vi "Message Handling Loop - File IO.vi"(8 "error in":errorcluster, 9 "Message Queues in":T1, 10 "User Event Bundle":T2) -> (0 "error out":errorcluster)   [LabVIEW 2018]
uses:
  Type Defs/User Events.ctl
  Support/Message Queue/All Message Queues.ctl
  Support/Message Queue/Message Cluster.ctl
  Type Defs/File IO Loop Data.ctl
  Type Defs/FGV States.ctl
  Support/Message Queue/Enqueue Message (Single).vi
  <vilib>/Utility/error.llb/Error Cluster From Error Code.vi
  <vilib>/ErrorRing/Error Ring.xnode
  Support/Message Queue/Message Queue.lvlib
  Support/User Events/User Events.lvlib
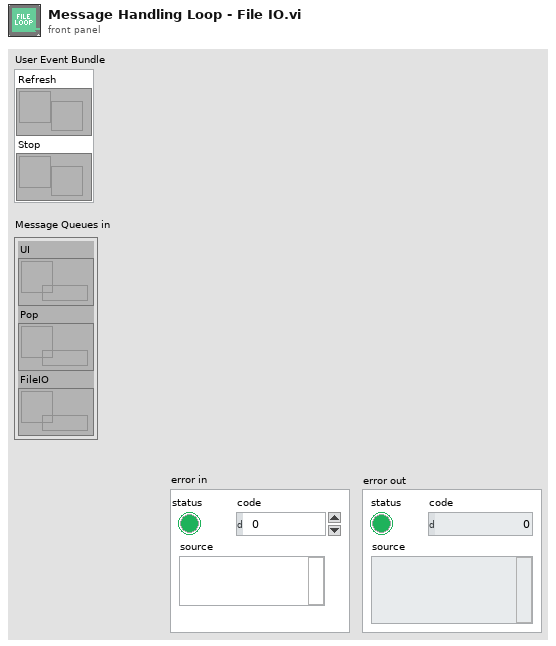
[diagram p1: front panel]
types:
  T1 = typedef "Message Queue.lvlib/All Message Queues.ctl" = cluster{"UI":refnum<queue>, "Pop":refnum<queue>, "FileIO":refnum<queue>}
  T2 = typedef "User Events.ctl" = cluster{"Refresh":refnum<user-event>, "Stop":refnum<user-event>}
  T3 = typedef "File IO Loop Data.ctl" = cluster{"Data Folder File Path":path, "UI":refnum<queue>, "Pop":refnum<queue>, "FileIO":refnum<queue>, "Open Notes":i32[], "Main VI":refnum<vi>, "Update Path":path}
  T4 = typedef "FGV States.ctl" = enum16{"Initialize", "Merge", "Write", "Remove", "Read", "Clear"}
  T5 = typedef "SR Cluster.ctl" = cluster{"Color":u32, "SR Number":i32, "SR Status":T6, "Name":string, "Summary":string, "Last Updated":timestamp, "SR Type":string, "Service Level":string, "Days Open":dbl, "Creation Date":timestamp, "Owner":string, "Note":string}
  T6 = typedef "SR Status.ctl" = enum16{"Caller Abandoned", "Created in Error", "Expired", "Forum Resolved AE", "Forum Resolved Customer", "IN WORK", "IN WORK Collab with AES", "IN WORK Collab with PSE", "IN WORK Collab with SE", "IN WORK Customer Added Note", "IN WORK Escalation", "IN WORK Wait on Customer", "Open", "Potentially Resolved", "Presumed Resolved", "RMA Approved for Return", "RMA Closed", "RMA Closed - DOA", "RMA In Progress", "RMA Open", "RMA Waiting on Customer", "Resolved", "Passed Off"}
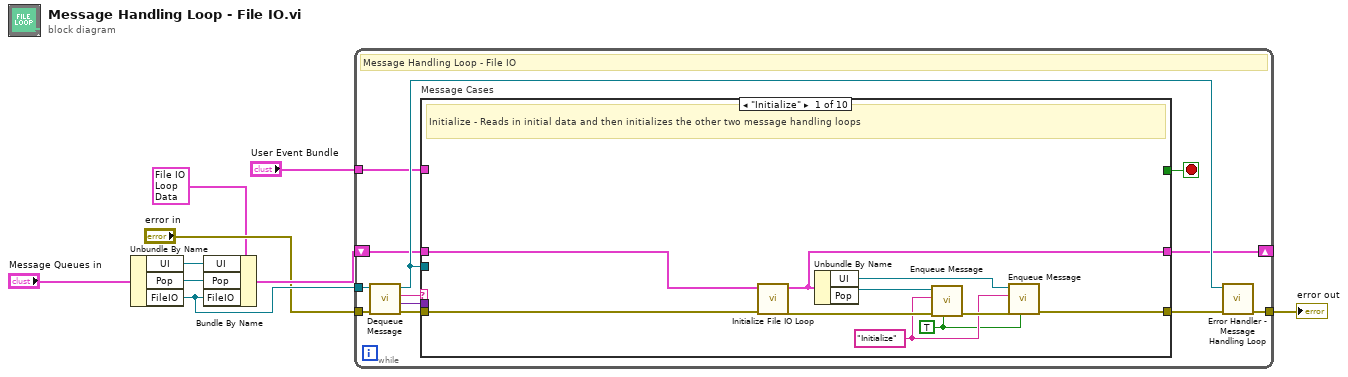
[diagram p0: block diagram]
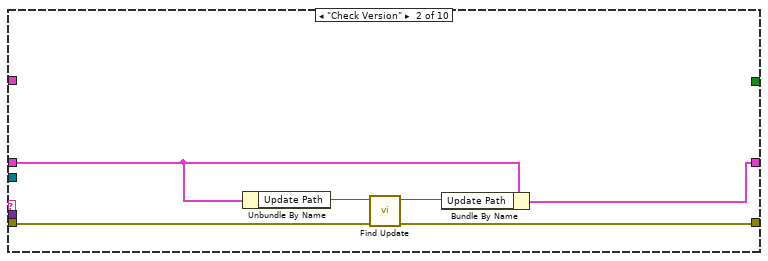
[diagram p2: hidden frame]
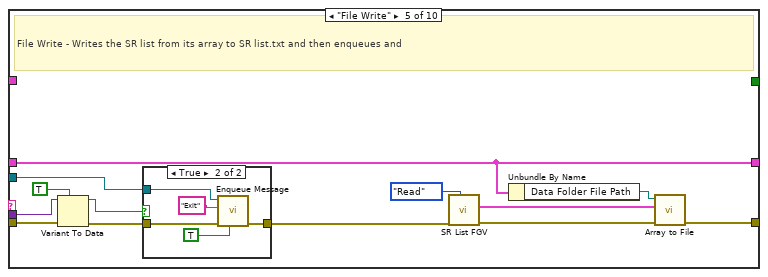
[diagram p5: hidden frame]
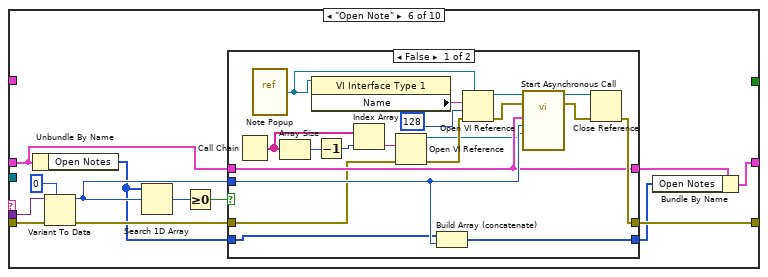
[diagram p7: hidden frame]
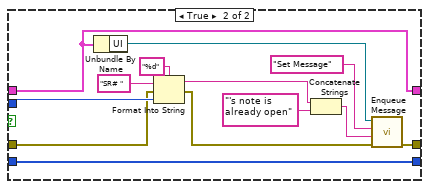
[diagram p8: hidden frame]
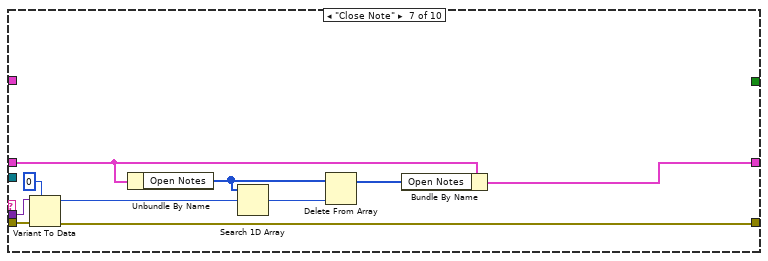
[diagram p9: hidden frame]
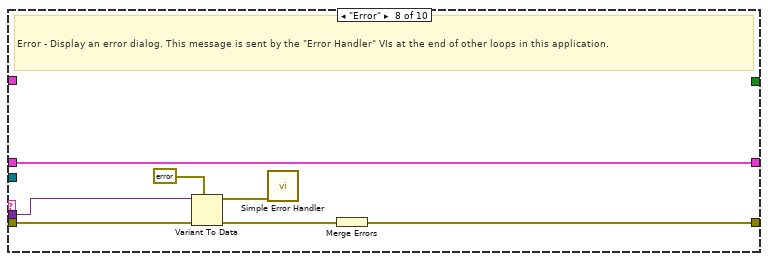
[diagram p10: hidden frame]
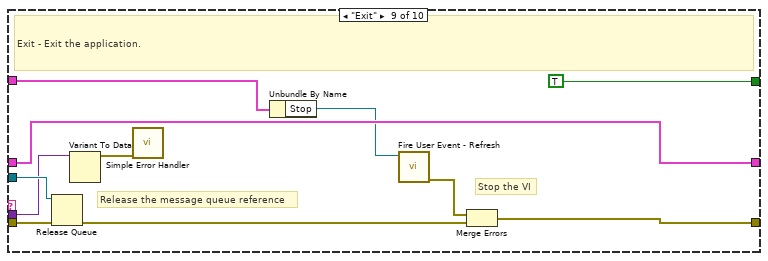
[diagram p11: hidden frame]
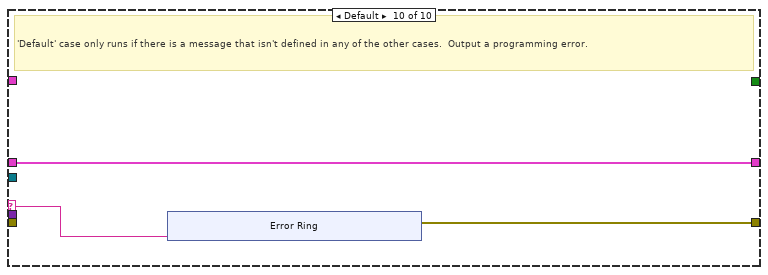
[diagram p12: hidden frame]
diagram:
  n1 = Unbundle By Name("Message Queues in") -> ("UI"=w6:refnum<queue>, "Pop"=w4:refnum<queue>, "FileIO"=w5:refnum<queue>)
  n2 = Bundle By Name(cluster=T3 {"Data Folder File Path"=path "", "UI"=refnum, "Pop"=refnum, "FileIO"=refnum, "Open Notes"=[], "Main VI"=refnum, "Update Path"=path ""} ("Data Loop Data"), "UI"=w6, "Pop"=w4, "FileIO"=w5) -> (w7:T3)
  n3 = while {
    tunnel: w5 -> [w17]
    tunnel: [w15] -> w1
    shift-right: [w12] -> _
    shift-left: w7 -> [w13]
    tunnel: "User Event Bundle" -> [w11]
    tunnel: "error in" -> [w10]
    stop <- w21 stop-if-true
    # "Message Handling Loop - File IO"
    n4 = call "Dequeue Message.vi"("error in (no error)"=w10, "Message Queue"=w17) -> ("error out"=w20:errorcluster, "Message Data"=w18:variant, "Message"=w19:string, "dup Message Queue"=w16:refnum<queue>)  [unwired: 6 in]
    n5 = case "Message Cases" shown="\"Initialize\"" w19 {
      selector: w19 -> [_ _ _ _ _ _ _ _ _ w135]
      tunnel: w16 -> [_ _ _ _ w46 _ _ _ w133 _]
      tunnel: w20 -> [w30 w37 w39 w41 w49 w72 w115 w122 w129 _]
      tunnel: [w25 w36 w39 w41 w50 w70 w112 w117 w130 w136] -> w14
      tunnel: [_ _ _ _ _ _ _ _ TRUE _] -> w21
      tunnel: w18 -> [_ _ _ _ w42 w73 w114 w121 w127 _]
      tunnel: w13 -> [w31 w34 w38 w40 w45 w64 w108 w116 w126 w134]
      tunnel: [w29 w32 w38 w40 w45 w61 w106 w116 w126 w134] -> w12
      tunnel: w11 -> [_ _ _ _ _ _ _ _ w125 _]
      frame "Initialize" {
        w22 = TRUE ("Priority Message? (F)")
        w23 = "Initialize" ("Message")
        # "Initialize - Reads in initial data and then initializes the other two message handling loops"
        n6 = call "Initialize File IO Loop.vi"("error in"=w30, "File Loop Data in"=w31) -> ("error out"=w24:errorcluster, "File Loop Data out"=w29:T3)  [unwired: 8 in]
        n7 = Unbundle By Name(w29) -> ("UI"=w27:refnum<queue>, "Pop"=w28:refnum<queue>)
        n8 = call-poly "Enqueue Message.vi"("Priority Message? (F)"=w22, "error in (no error)"=w24, "Message"=w23, "Message Queue"=w28) -> ("error out"=w26:errorcluster)  [unwired: 6 in, 1 out]
        n9 = call-poly "Enqueue Message.vi"("Priority Message? (F)"=w22, "error in (no error)"=w26, "Message"=w23, "Message Queue"=w27) -> ("error out"=w25:errorcluster)  [unwired: 6 in, 1 out]
      }
      frame "Check Version" {
        n10 = Unbundle By Name(w34) -> ("Update Path"=w35:path)
        n11 = call "Find Update.vi"("Error In"=w37, "search path"=w35) -> ("Error Out"=w36:errorcluster, "update path"=w33:path)  [unwired: 6 in, 2 out]
        n12 = Bundle By Name(cluster=w34, "Update Path"=w33) -> (w32:T3)
      }
      frame "Download Update" {
      }
      frame "Install Update" {
      }
      frame "File Write" {
        # "File Write - Writes the SR list from its array to SR list.txt and then enqueues and"
        n13 = Variant To Data(error in=w49, type=TRUE ("Priority Message? (F)"), Variant=w42) -> (data=w44:bool, error out=w48:errorcluster)
        n14 = case shown="True" w44 {
          tunnel: w48 -> [w55 w58]
          tunnel: [w55 w57] -> w47
          tunnel: w46 -> [_ w56]
          frame False {
          }
          frame True {
            n15 = call-poly "Enqueue Message.vi"("Priority Message? (F)"=TRUE, "error in (no error)"=w58, "Message"="Exit", "Message Queue"=w56) -> ("error out"=w57:errorcluster)  [unwired: 6 in, 1 out]
          }
        }
        n16 = call "SR List FGV.vi"("Operation"=FGV_States."Read", "Error In"=w47) -> ("Error Out"=w54:errorcluster, "list out"=w52:T5[])  [unwired: 8 in]
        n17 = Unbundle By Name(w45) -> ("Data Folder File Path"=w51:path)
        n18 = call "Array to File.vi"("error in"=w54, "array in"=w52, "file path in"=w51) -> ("error out"=w50:errorcluster)  [unwired: 7 in, 1 out]
      }
      frame "Open Note" {
        n19 = Unbundle By Name(w64) -> ("Open Notes"=w65:i32[])
        n20 = Variant To Data(error in=w72, type=0, Variant=w73) -> (data=w68:i32, error out=w69:errorcluster)
        n21 = Search 1D Array(1D array=w65, element=w68) -> (index of element=w66:i32)  [unwired: 1 in]
        n22 = Greater Or Equal To 0?(x=w66) -> (x >= 0?=w67:bool)
        n23 = case shown="False" w67 {
          tunnel: [w92 w104] -> w70
          tunnel: w64 -> [w81 w93]
          tunnel: w69 -> [w76 w97]
          tunnel: w68 -> [w85 w101]
          tunnel: w65 -> [w82 w105]
          tunnel: [w84 w105] -> w62
          tunnel: [w81 w93] -> w63
          frame False {
            n24 = Call Chain() -> (call chain=w80:string[])
            n25 = vi-ref "Note Popup.vi"() -> (w83:refnum<vi>)
            n26 = Array Size(array=w80) -> (size(s)=w77:i32)
            n27 = property class="VI Interface Type 1"(reference=w83) -> ("Name"=w91:string)  [unwired: 1 in, 2 out]
            n28 = Decrement(x=w77) -> (x-1=w79:i32)
            n29 = Index Array(array=w80, index=w79) -> (element=w78:string)
            n30 = Open VI Reference(vi path=w78, error in (no error)=w76) -> (vi reference=w74:refnum<vi>, error out=w75:errorcluster)  [unwired: 4 in]
            n31 = Build Array (concatenate)(w82, w85) -> (w84:i32[])
            n32 = Open VI Reference(type specifier VI Refnum (for type only)=w83, vi path=w91, options=128, error in (no error)=w75) -> (vi reference=w87:refnum<vi>, error out=w86:errorcluster)  [unwired: 2 in]
            n33 = call-by-ref "Start Asynchronous Call"(reference=w87, error in=w86, "Main VI ref"=w74, "SR Number"=w85, "File Loop Data"=w81) -> (reference out=w90:refnum<vi>, error out=w89:errorcluster)  [unwired: 9 in]
            n34 = Close Reference(reference=w90, error in (no error)=w89) -> (error out=w92:errorcluster)
          }
          frame True {
            n35 = Unbundle By Name(w93) -> ("UI"=w103:refnum<queue>)
            n36 = Format Into String(format string="%d", initial string="SR# ", error in=w97, w101) -> (resulting string=w99:string, error out=w98:errorcluster)
            n37 = Concatenate Strings(w99, "'s note is already open" ("string")) -> (w95:string)
            n38 = call-poly "Enqueue Message.vi"("error in (no error)"=w98, "Message Data"=w95, "Message"="Set Message", "Message Queue"=w103) -> ("error out"=w104:errorcluster)  [unwired: 6 in, 1 out]
          }
        }
        n39 = Bundle By Name(cluster=w63, "Open Notes"=w62) -> (w61:T3)
      }
      frame "Close Note" {
        n40 = Variant To Data(error in=w115, type=0, Variant=w114) -> (data=w111:i32, error out=w112:errorcluster)
        n41 = Unbundle By Name(w108) -> ("Open Notes"=w109:i32[])
        n42 = Search 1D Array(1D array=w109, element=w111) -> (index of element=w110:i32)  [unwired: 1 in]
        n43 = Delete From Array(array=w109, index=w110) -> (array with subset deleted=w107:i32[])  [unwired: 1 in, 1 out]
        n44 = Bundle By Name(cluster=w108, "Open Notes"=w107) -> (w106:T3)
      }
      frame "Error" {
        # "Error - Display an error dialog. This message is sent by the \"Error Handler\" VIs at the end of other loops in this application."
        n45 = Variant To Data(error in=w122, type=errorcluster {"status"=FALSE, "code"=0, "source"=""} ("error constant"), Variant=w121) -> (data=w119:errorcluster, error out=w118:errorcluster)
        n46 = call <vilib>:"Simple Error Handler.vi"("error in (no error)"=w119) -> ()  [unwired: 4 in, 5 out]
        n47 = Merge Errors(w118) -> (w117:errorcluster)
      }
      frame "Exit" {
        # "Stop the VI"
        # "Release the message queue reference"
        # "Exit - Exit the application."
        n48 = Release Queue(queue=w133, error in (no error)=w129) -> (error out=w131:errorcluster)  [unwired: 1 in, 2 out]
        n49 = Variant To Data(Variant=w127) -> (data=w128:errorcluster)  [unwired: 2 in, 1 out]
        n50 = call <vilib>:"Simple Error Handler.vi"("error in (no error)"=w128) -> ()  [unwired: 4 in, 5 out]
        n51 = Unbundle By Name(w125) -> ("Stop"=w124:refnum<user-event>)
        n52 = call "Fire User Event - Refresh.vi"("Refresh"=w124) -> ("error out"=w123:errorcluster)  [unwired: 10 in]
        n53 = Merge Errors(w123, w131) -> (w130:errorcluster)
      }
      frame Default {
        # "'Default' case only runs if there is a message that isn't defined in any of the other cases.  Output a programming error."
        n54 = xnode "Error Ring"("parameter 0"=w135) -> ("error out"=w136:errorcluster)
      }
    }
    n55 = call "Error Handler - Message Handling Loop.vi"("error in (no error)"=w14, "Message Queue"=w16) -> ("dup error in"=w15:errorcluster)  [unwired: 8 in, 1 out]
  }
  "error out" <- w1
